vi "GetAutoInTeleop.vi"(1 "AutoInTeleopOverride":bool) -> (0 "AutoInTeleop":bool)   [LabVIEW 2017]
uses:
  <vilib>/Rock Robotics/Network Tables/NT Read Boolean.vi
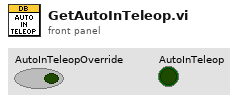
[diagram p1: front panel]
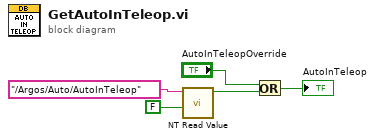
[diagram p0: block diagram]
diagram:
  n1 = call-poly <vilib>:"NT Read Value.vi"("Default Value"=FALSE, "Name"="/Argos/Auto/AutoInTeleop") -> ("Boolean"=w3:bool)  [unwired: 8 in, 1 out]
  n2 = Or(x="AutoInTeleopOverride", y=w3) -> (x .or. y?=→"AutoInTeleop":bool)
